vi "FM Set Offset.vi"(0 "Offset (V)":dbl format="%.1f") -> ()   [LabVIEW 2019]
uses:
  MWC Global.vi
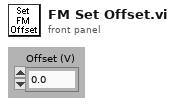
[diagram p1: front panel]
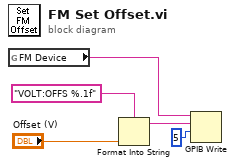
[diagram p0: block diagram]
diagram:
  n1 = global read "MWC Global.vi" "FM Device"() -> (w3:string)
  n2 = Format Into String(format string="VOLT:OFFS %.1f" ("Format String"), "Offset (V)") -> (resulting string=w5:string)  [unwired: 2 in, 1 out]
  n3 = GPIB Write(0:w3, 1:w5, 2:i16 5 ("mode (0)")) -> ()  [unwired: 2 in, 2 out]
